vi "Point To Hub.vi"(10 "Input Velocities":T1) -> (2 "omega":dbl format="%.2f")   [LabVIEW 2025]
uses:
  swerve-template/Type Definitions/Data/Robot Velocities.ctl
  <vilib>/Analysis/coordinate.llb/Angle Units.ctl
  <vilib>/Analysis/coordinate.llb/Angle Range (Degree).ctl
  <vilib>/Analysis/coordinate.llb/Wrap Angle (scalar).vi
  <vilib>/Rock Robotics/Network Tables/NT Read Number.vi
  <vilib>/Rock Robotics/Network Tables/NT Read Numeric Array.vi
  <vilib>/addons/control/pid/pid.llb/PID (DBL).vi
  <vilib>/Analysis/NI_AAL_Angle.lvlib
  <vilib>/addons/control/pid/NI_PID_pid.lvlib
panel:
  in  "TOF":dbl
  in  "tolerance":dbl=2.0
  in  "F term":dbl=1.7
  out "Waveform Chart":cluster{"angle out":dbl, "Numeric":dbl}(graph)
  out "angle out":dbl
  out "error":dbl
  in  "PID gains":T2={"proportional gain (Kc)"=4.8, "integral time (Ti, min)"=0.0, "derivative time (Td, min)"=0.0}
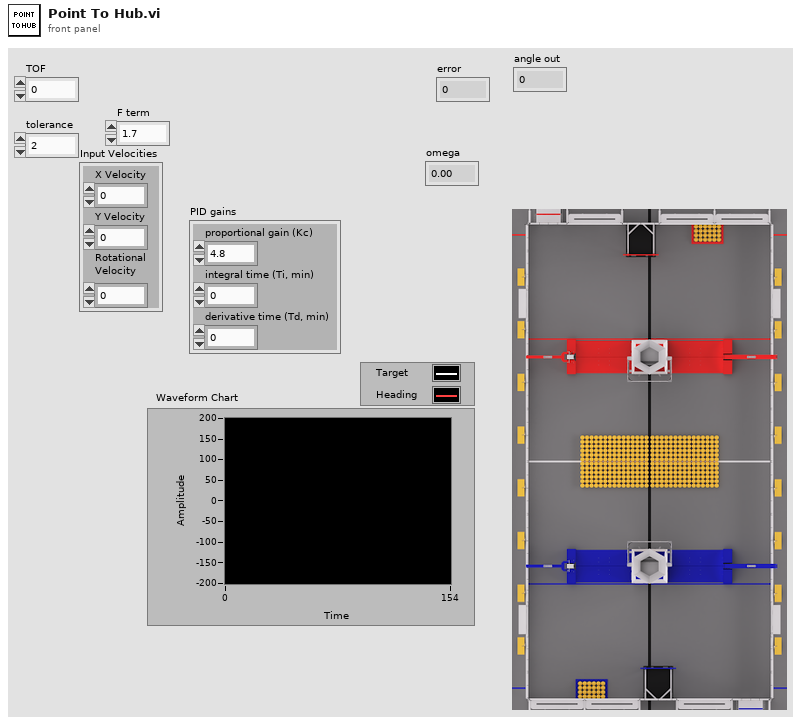
[diagram p1: front panel]
types:
  T1 = typedef "Robot Velocities.ctl" = cluster{"X Velocity":dbl, "Y Velocity":dbl, "Rotational \nVelocity":dbl}
  T2 = cluster{"proportional gain (Kc)":dbl, "integral time (Ti, min)":dbl, "derivative time (Td, min)":dbl}
  T3 = typedef "NI_AAL_Angle.lvlib/Angle Units.ctl" = i32
  T4 = typedef "NI_AAL_Angle.lvlib/Angle Range (Degree).ctl" = u16
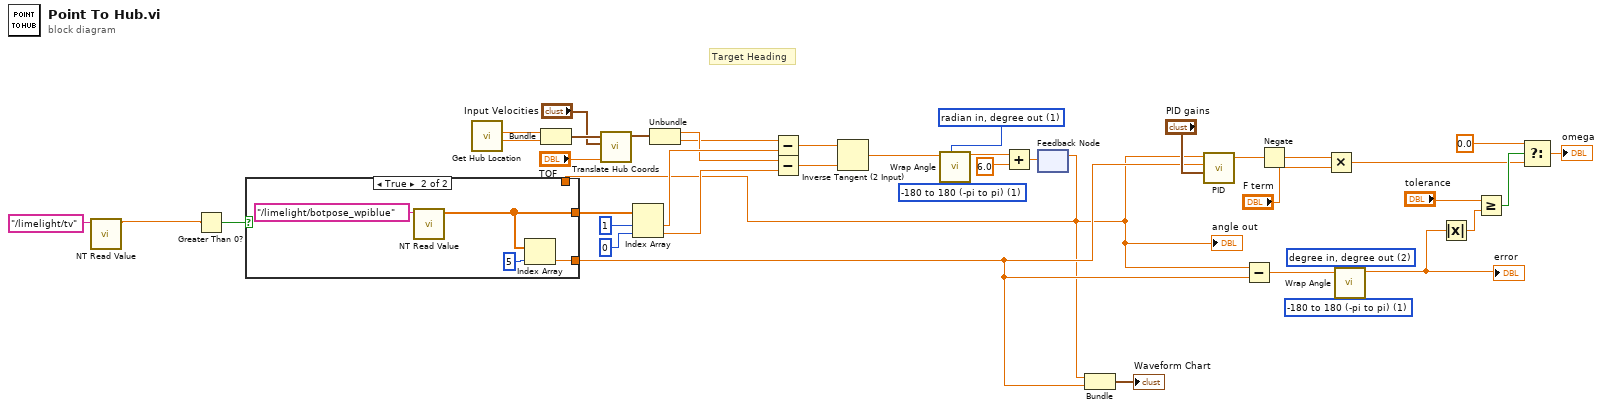
[diagram p0: block diagram]
diagram:
  w28 = T3 1 items=["radian in, radian out", "radian in, degree out", "degree in, degree out", "degree in, radian out"] ("angle units")
  w33 = T4 1 items=["none", "-180 to 180 (-pi to pi)", "0 to 360 (0 to 2pi)"] ("angle range")
  w34 = T3 2 items=["radian in, radian out", "radian in, degree out", "degree in, degree out", "degree in, radian out"] ("angle units")
  w40 = T4 1 items=["none", "-180 to 180 (-pi to pi)", "0 to 360 (0 to 2pi)"] ("angle range")
  # "Target Heading"
  n1 = call-poly <vilib>:"NT Read Value.vi"("name"="/limelight/tv") -> ("value"=w31:dbl)  [unwired: 8 in, 2 out]
  n2 = Greater Than 0?(x=w31) -> (x > 0?=w30:bool)
  n3 = call "Get Hub Location.vi"() -> ("Hub Y"=w5:dbl, "Hub X"=w6:dbl)  [unwired: 10 in]
  n4 = Bundle("Hub X"=w6, "Hub Y"=w5) -> (w8:cluster{"Hub X":dbl, "Hub Y":dbl})  [unwired: 1 in]
  n5 = call "Translate Hub Coords.vi"("TOF"="TOF", "Input Velocities"="Input Velocities", "Hub Coords"=w8) -> ("Hub Coords Out"=w7:cluster{"X":dbl, "Y":dbl})  [unwired: 6 in, 2 out]
  n6 = Unbundle(w7) -> ("X"=w4:dbl, "Y"=w3:dbl)
  n7 = feedback #1() -> (w10:dbl)  [unwired: 1 in]
  "angle out" <- w10
  n8 = case shown="True" w30 {
    tunnel: [_ w45] -> w25
    tunnel: [w42 w43] -> w12
    tunnel: w10 -> [w42 _]
    frame False {
    }
    frame True {
      n9 = call-poly <vilib>:"NT Read Value.vi"("name"="/limelight/botpose_wpiblue") -> ("value"=w45:dbl[])  [unwired: 8 in, 2 out]
      n10 = Index Array(array=w45, index=5) -> (element=w43:dbl)
    }
  }
  n11 = Index Array(array=w25, index #1=1 ("index"), index #2=0 ("index")) -> (element #1=w27:dbl, element #2=w26:dbl)
  n12 = Subtract(x=w3, y=w27) -> (x-y=w36:dbl)
  n13 = Subtract(x=w4, y=w26) -> (x-y=w37:dbl)
  n14 = Inverse Tangent (2 Input)(1:w37, 2:w36) -> (0:w24:dbl)
  n15 = call-poly <vilib>:"Wrap Angle.vi"("angle units"=w28, "angle range"=w40, "angle in"=w24) -> ("angle out"=w20:dbl)  [unwired: 7 in, 1 out]
  n16 = Add(x=w20, y=6.0) -> (x+y=w11:dbl)
  n17 = feedback-in #1(w11) -> ()
  n18 = Bundle(w10, "Numeric"=w12) -> (→"Waveform Chart":cluster{dbl, "Numeric":dbl})  [unwired: 1 in]
  n19 = call-poly <vilib>:"PID.vi"("PID gains"="PID gains", "process variable"=w12, "setpoint"=w10) -> ("output"=w38:dbl)  [unwired: 7 in, 1 out]
  n20 = Subtract(x=w10, y=w12) -> (x-y=w35:dbl)
  n21 = Negate(x=w38) -> (-x=w22:dbl)
  n22 = Multiply(x=w22, y="F term") -> (x*y=w9:dbl)
  n23 = call-poly <vilib>:"Wrap Angle.vi"("angle units"=w34, "angle range"=w33, "angle in"=w35) -> ("angle out"=w15:dbl)  [unwired: 7 in, 1 out]
  "error" <- w15
  n24 = Absolute Value(x=w15) -> (abs(x)=w14:dbl)
  n25 = Greater Or Equal?(x="tolerance", y=w14) -> (x >= y?=w16:bool)
  n26 = Select(t=0.0, s=w16, f=w9) -> (s? t:f=→"omega":dbl)
